vi "DeleteOldTargets.vi"(1 "TargetsIn":T1[](array[typedef])=[{"Target Type"=0, "Checksum"=0, "Signature Number"=0, "X Center"=0, "Y Center"=0, "Width"=0, "Height"=0, "Angle"=0}] {"Angle" format="%x"; "Height" format="%x"; "Width" format="%x"; "Y Center" format="%x"; "X Center" format="%x"; "Signature Number" format="%x"; "Checksum" format="%x"; "Target Type" items=["PIXY_START_WORD"=43605, "PIXY_START_WORD_CC"=43606, "PIXY_START_WORDX"=21930]}) -> (0 "TargetsOut":T1[](array[typedef]) {"Angle" format="%x"; "Height" format="%x"; "Width" format="%x"; "Y Center" format="%x"; "X Center" format="%x"; "Signature Number" format="%x"; "Checksum" format="%x"; "Target Type" items=["PIXY_START_WORD"=43605, "PIXY_START_WORD_CC"=43606, "PIXY_START_WORDX"=21930]})   [LabVIEW 2016, in "PixyCam_LabVIEW.lvlib"]
uses:
  PixyCam_LabVIEW.lvlib
  PixyCam_TargetData.ctl
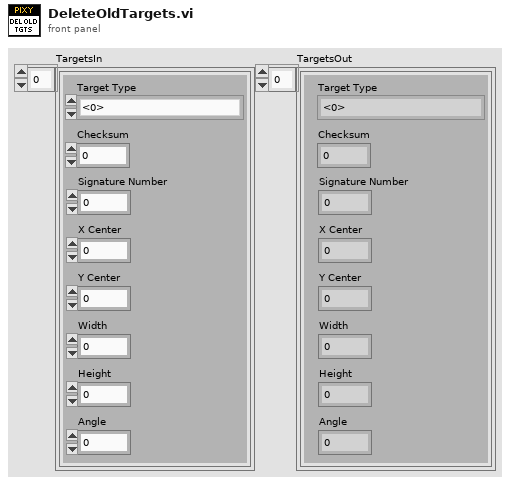
[diagram p1: front panel]
types:
  T1 = typedef "PixyCam_LabVIEW.lvlib/PixyCam_TargetData.ctl" = cluster{"Target Type":u16, "Checksum":u16, "Signature Number":u16, "X Center":u16, "Y Center":u16, "Width":u16, "Height":u16, "Angle":u16}
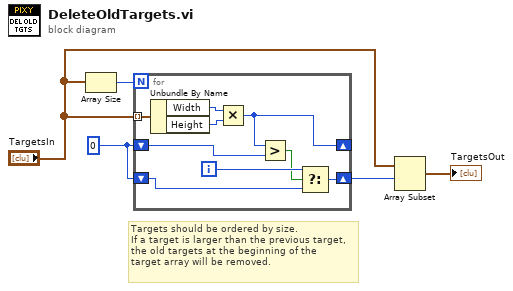
[diagram p0: block diagram]
diagram:
  w5 = u16 0
  # "Targets should be ordered by size.\nIf a target is larger than the previous target,\nthe old targets at the beginning of the\ntarget array will be removed."
  n1 = Array Size(array="TargetsIn") -> (size(s)=w1:i32)
  n2 = for {
    N: w1 -> [_]
    tunnel: "TargetsIn" -> [w14] mode=indexing
    shift-right: [w8] -> _
    shift-left: w5 -> [w7]
    shift-right: [w10] -> w2
    shift-left: w5 -> [w6]
    i -> [w11]
    n3 = Unbundle By Name(w14) -> ("Width"=w13:u16, "Height"=w12:u16)
    n4 = Multiply(x=w13, y=w12) -> (x*y=w8:u16)
    n5 = Greater?(x=w8, y=w7) -> (0:w9:bool)
    n6 = Select(t=w11, s=w9, f=w6) -> (s? t:f=w10:i32)
  }
  n7 = Array Subset(array="TargetsIn", index=w2) -> (→"TargetsOut":T1[])  [unwired: 1 in]
